vi "Format String to Numeric.vi"(0 "Expected String":string, 1 "Data Parameters.List":string[](array[string]), 2 "Ignore String":string, 5 "Format String":string, 7 "Endian":T1, 9 "Channel Type":T2, 11 "error in (no error)":errorcluster, 12 "Type":T3, 13 "Response":string) -> (4 "remaining string":string, 6 "Value":dbl, 15 "error out":errorcluster)   [LabVIEW 2020, in "Instrument Addon Engine.lvlib"]
uses:
  Instrument Addon Engine.lvlib
  Addon Shared/Types/Type Cast Type.ctl
  Addon Shared/Types/Data Channel Type.ctl
  Addon Shared/Types/Endian.ctl
  Addon Shared/Instrument Addon Shared.lvlib
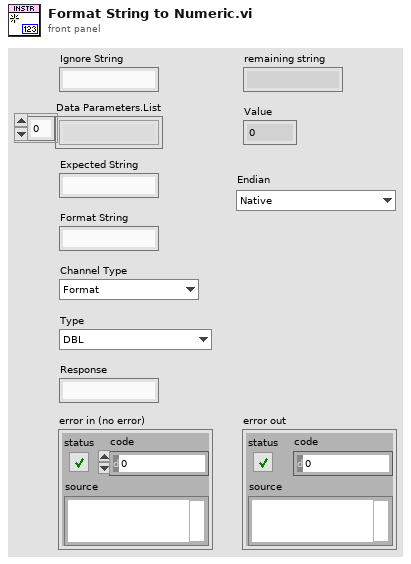
[diagram p1: front panel]
types:
  T1 = typedef "Instrument Addon Shared.lvlib/Endian.ctl" = enum16{"Native", "Little", "Big"}
  T2 = typedef "Instrument Addon Shared.lvlib/Data Channel Type.ctl" = enum16{"Format", "Comparison", "Type Cast", "Enumerated List"}
  T3 = typedef "Instrument Addon Shared.lvlib/Type Cast Type.ctl" = enum16{"DBL", "SGL", "U64", "U32", "U16", "U8", "I64", "I32", "I16", "I8"}
  T4 = enum16{"big-endian, network order", "native, host order", "little-endian"}
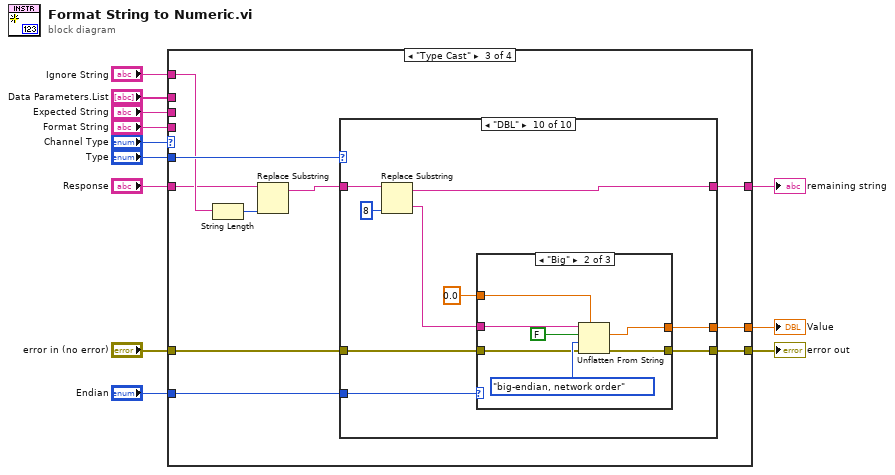
[diagram p0: block diagram]
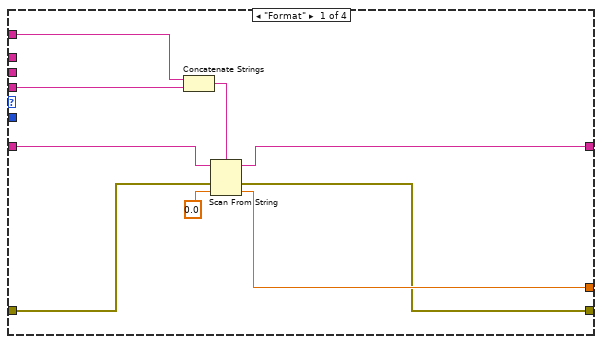
[diagram p2: hidden frame]
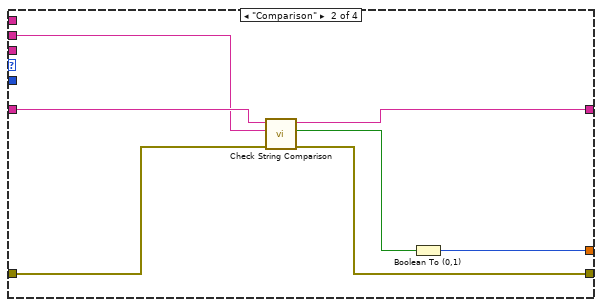
[diagram p3: hidden frame]
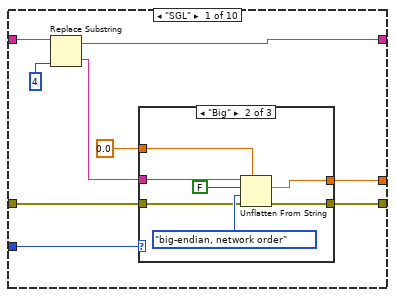
[diagram p4: hidden frame]
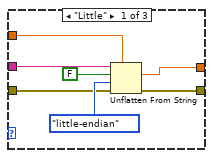
[diagram p5: hidden frame]
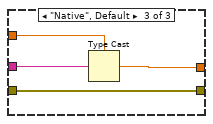
[diagram p6: hidden frame]
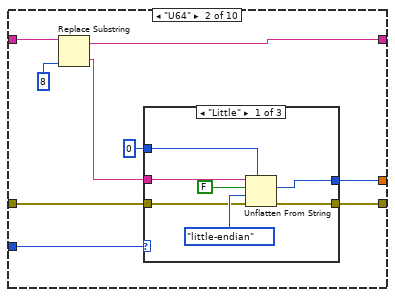
[diagram p7: hidden frame]
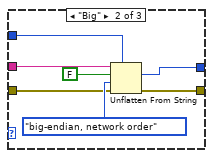
[diagram p8: hidden frame]
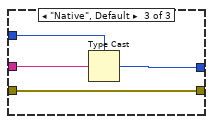
[diagram p9: hidden frame]
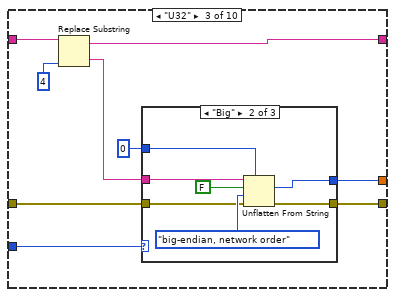
[diagram p10: hidden frame]
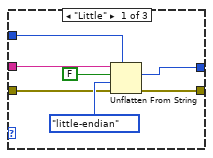
[diagram p11: hidden frame]
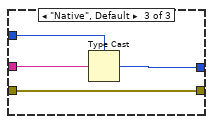
[diagram p12: hidden frame]
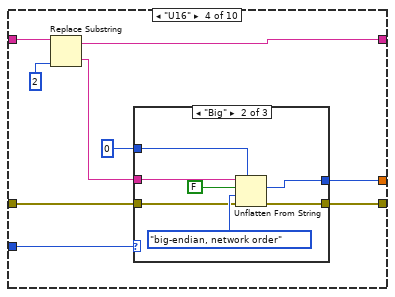
[diagram p13: hidden frame]
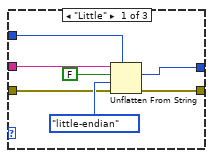
[diagram p14: hidden frame]
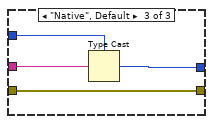
[diagram p15: hidden frame]
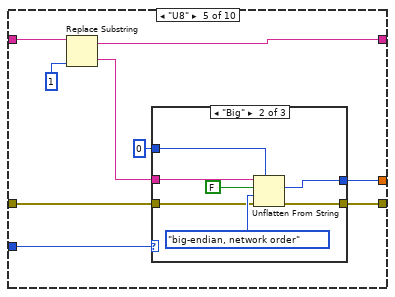
[diagram p16: hidden frame]
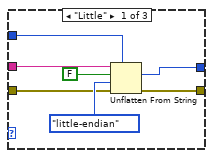
[diagram p17: hidden frame]
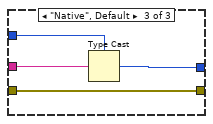
[diagram p18: hidden frame]
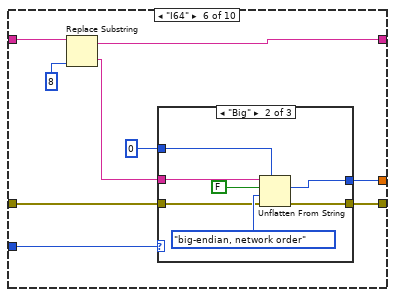
[diagram p19: hidden frame]
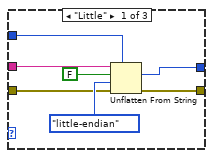
[diagram p20: hidden frame]
diagram:
  n1 = case shown="\"Type Cast\"" "Channel Type" {
    tunnel: [w20 w28 w37 w315] -> w10
    tunnel: "Response" -> [w21 w27 w34 w310]
    tunnel: [w19 w25 w38 w313] -> w4
    tunnel: "Ignore String" -> [w17 _ w35 w311]
    tunnel: "Format String" -> [w16 _ _ _]
    tunnel: "error in (no error)" -> [w15 w23 w32 w317]
    tunnel: [w14 w22 w29 w314] -> w7
    tunnel: "Expected String" -> [_ w26 _ _]
    tunnel: "Type" -> [_ _ w36 _]
    tunnel: "Data Parameters.List" -> [_ _ _ w316]
    tunnel: "Endian" -> [_ _ w30 _]
    frame "Format" {
      n2 = Concatenate Strings(w17, w16) -> (w13:string)
      n3 = Scan From String(format string=w13, input string=w21, error in=w15, default 1=0.0 ("default value 1")) -> (remaining string=w19:string, error out=w14:errorcluster, output 1=w20:dbl)  [unwired: 1 in, 1 out]
    }
    frame "Comparison" {
      n4 = call "Check String Comparison.vi"("error in (no error)"=w23, "Expected String"=w26, "String"=w27) -> ("error out"=w22:errorcluster, "Found?"=w24:bool, "string out"=w25:string)  [unwired: 6 in]
      n5 = Boolean To (0,1)(Boolean=w24) -> (0, 1=w28:i16)
    }
    frame "Type Cast" {
      n6 = String Length(string=w35) -> (length=w31:i32)
      n7 = Replace Substring(2:w31, 5:w34) -> (1:w33:string)  [unwired: 2 in, 1 out]
      n8 = case shown="\"DBL\"" w36 {
        tunnel: w33 -> [w47 w74 w101 w128 w155 w182 w209 w236 w263 w290]
        tunnel: [w46 w73 w100 w127 w154 w181 w208 w235 w262 w289] -> w38
        tunnel: [w39 w67 w93 w122 w147 w174 w202 w229 w259 w282] -> w37
        tunnel: w32 -> [w42 w70 w98 w125 w152 w179 w206 w230 w256 w287]
        tunnel: w30 -> [w41 w66 w95 w124 w151 w178 w201 w228 w258 w285]
        tunnel: [w40 w71 w94 w123 w148 w175 w203 w233 w255 w286] -> w29
        frame "SGL" {
          n9 = Replace Substring(2:4 ("length (len. of substring)"), 5:w47) -> (0:w44:string, 1:w46:string)  [unwired: 2 in]
          n10 = case shown="\"Big\"" w41 {
            tunnel: w44 -> [w54 w61 w65]
            tunnel: [w50 w57 w64] -> w39
            tunnel: sgl 0.0 -> [w51 w58 w63]
            tunnel: w42 -> [w49 w56 w62]
            tunnel: [w48 w55 w62] -> w40
            frame "Little" {
              n11 = Unflatten From String(type=w51, binary string=w54, data includes array or string size? (T)=FALSE, byte order (0:big-endian, network order)=T4."little-endian", error in (no error)=w49) -> (value=w50:sgl, error out=w48:errorcluster)  [unwired: 1 out]
            }
            frame "Big" {
              n12 = Unflatten From String(type=w58, binary string=w61, data includes array or string size? (T)=FALSE, byte order (0:big-endian, network order)=T4."big-endian, network order", error in (no error)=w56) -> (value=w57:sgl, error out=w55:errorcluster)  [unwired: 1 out]
            }
            frame "Native", Default {
              n13 = Type Cast(type=w63, x=w65) -> (*(type *) &x=w64:sgl)
            }
          }
        }
        frame "U64" {
          n14 = Replace Substring(2:8 ("length (len. of substring)"), 5:w74) -> (0:w69:string, 1:w73:string)  [unwired: 2 in]
          n15 = case shown="\"Little\"" w66 {
            tunnel: w69 -> [w81 w88 w92]
            tunnel: [w77 w84 w91] -> w67
            tunnel: u64 0 -> [w78 w85 w90]
            tunnel: w70 -> [w76 w83 w89]
            tunnel: [w75 w82 w89] -> w71
            frame "Little" {
              n16 = Unflatten From String(type=w78, binary string=w81, data includes array or string size? (T)=FALSE, byte order (0:big-endian, network order)=T4."little-endian", error in (no error)=w76) -> (value=w77:u64, error out=w75:errorcluster)  [unwired: 1 out]
            }
            frame "Big" {
              n17 = Unflatten From String(type=w85, binary string=w88, data includes array or string size? (T)=FALSE, byte order (0:big-endian, network order)=T4."big-endian, network order", error in (no error)=w83) -> (value=w84:u64, error out=w82:errorcluster)  [unwired: 1 out]
            }
            frame "Native", Default {
              n18 = Type Cast(type=w90, x=w92) -> (*(type *) &x=w91:u64)
            }
          }
        }
        frame "U32" {
          n19 = Replace Substring(2:4 ("length (len. of substring)"), 5:w101) -> (0:w97:string, 1:w100:string)  [unwired: 2 in]
          n20 = case shown="\"Big\"" w95 {
            tunnel: w97 -> [w108 w115 w119]
            tunnel: [w104 w111 w118] -> w93
            tunnel: u32 0 -> [w105 w112 w117]
            tunnel: w98 -> [w103 w110 w116]
            tunnel: [w102 w109 w116] -> w94
            frame "Little" {
              n21 = Unflatten From String(type=w105, binary string=w108, data includes array or string size? (T)=FALSE, byte order (0:big-endian, network order)=T4."little-endian", error in (no error)=w103) -> (value=w104:u32, error out=w102:errorcluster)  [unwired: 1 out]
            }
            frame "Big" {
              n22 = Unflatten From String(type=w112, binary string=w115, data includes array or string size? (T)=FALSE, byte order (0:big-endian, network order)=T4."big-endian, network order", error in (no error)=w110) -> (value=w111:u32, error out=w109:errorcluster)  [unwired: 1 out]
            }
            frame "Native", Default {
              n23 = Type Cast(type=w117, x=w119) -> (*(type *) &x=w118:u32)
            }
          }
        }
        frame "U16" {
          n24 = Replace Substring(2:2 ("length (len. of substring)"), 5:w128) -> (0:w120:string, 1:w127:string)  [unwired: 2 in]
          n25 = case shown="\"Big\"" w124 {
            tunnel: w120 -> [w135 w142 w146]
            tunnel: [w131 w138 w145] -> w122
            tunnel: u16 0 -> [w132 w139 w144]
            tunnel: w125 -> [w130 w137 w143]
            tunnel: [w129 w136 w143] -> w123
            frame "Little" {
              n26 = Unflatten From String(type=w132, binary string=w135, data includes array or string size? (T)=FALSE, byte order (0:big-endian, network order)=T4."little-endian", error in (no error)=w130) -> (value=w131:u16, error out=w129:errorcluster)  [unwired: 1 out]
            }
            frame "Big" {
              n27 = Unflatten From String(type=w139, binary string=w142, data includes array or string size? (T)=FALSE, byte order (0:big-endian, network order)=T4."big-endian, network order", error in (no error)=w137) -> (value=w138:u16, error out=w136:errorcluster)  [unwired: 1 out]
            }
            frame "Native", Default {
              n28 = Type Cast(type=w144, x=w146) -> (*(type *) &x=w145:u16)
            }
          }
        }
        frame "U8" {
          n29 = Replace Substring(2:1 ("length (len. of substring)"), 5:w155) -> (0:w150:string, 1:w154:string)  [unwired: 2 in]
          n30 = case shown="\"Big\"" w151 {
            tunnel: w150 -> [w162 w169 w173]
            tunnel: [w158 w165 w172] -> w147
            tunnel: u8 0 -> [w159 w166 w171]
            tunnel: w152 -> [w157 w164 w170]
            tunnel: [w156 w163 w170] -> w148
            frame "Little" {
              n31 = Unflatten From String(type=w159, binary string=w162, data includes array or string size? (T)=FALSE, byte order (0:big-endian, network order)=T4."little-endian", error in (no error)=w157) -> (value=w158:u8, error out=w156:errorcluster)  [unwired: 1 out]
            }
            frame "Big" {
              n32 = Unflatten From String(type=w166, binary string=w169, data includes array or string size? (T)=FALSE, byte order (0:big-endian, network order)=T4."big-endian, network order", error in (no error)=w164) -> (value=w165:u8, error out=w163:errorcluster)  [unwired: 1 out]
            }
            frame "Native", Default {
              n33 = Type Cast(type=w171, x=w173) -> (*(type *) &x=w172:u8)
            }
          }
        }
        frame "I64" {
          n34 = Replace Substring(2:8 ("length (len. of substring)"), 5:w182) -> (0:w177:string, 1:w181:string)  [unwired: 2 in]
          n35 = case shown="\"Big\"" w178 {
            tunnel: w177 -> [w189 w196 w200]
            tunnel: [w185 w192 w199] -> w174
            tunnel: i64 0 -> [w186 w193 w198]
            tunnel: w179 -> [w184 w191 w197]
            tunnel: [w183 w190 w197] -> w175
            frame "Little" {
              n36 = Unflatten From String(type=w186, binary string=w189, data includes array or string size? (T)=FALSE, byte order (0:big-endian, network order)=T4."little-endian", error in (no error)=w184) -> (value=w185:i64, error out=w183:errorcluster)  [unwired: 1 out]
            }
            frame "Big" {
              n37 = Unflatten From String(type=w193, binary string=w196, data includes array or string size? (T)=FALSE, byte order (0:big-endian, network order)=T4."big-endian, network order", error in (no error)=w191) -> (value=w192:i64, error out=w190:errorcluster)  [unwired: 1 out]
            }
            frame "Native", Default {
              n38 = Type Cast(type=w198, x=w200) -> (*(type *) &x=w199:i64)
            }
          }
        }
        frame "I32" {
          n39 = Replace Substring(2:4 ("length (len. of substring)"), 5:w209) -> (0:w205:string, 1:w208:string)  [unwired: 2 in]
          n40 = case shown="\"Native\", Default" w201 {
            tunnel: w205 -> [w216 w223 w227]
            tunnel: [w212 w219 w226] -> w202
            tunnel: 0 -> [w213 w220 w225]
            tunnel: w206 -> [w211 w218 w224]
            tunnel: [w210 w217 w224] -> w203
            frame "Little" {
              n41 = Unflatten From String(type=w213, binary string=w216, data includes array or string size? (T)=FALSE, byte order (0:big-endian, network order)=T4."little-endian", error in (no error)=w211) -> (value=w212:i32, error out=w210:errorcluster)  [unwired: 1 out]
            }
            frame "Big" {
              n42 = Unflatten From String(type=w220, binary string=w223, data includes array or string size? (T)=FALSE, byte order (0:big-endian, network order)=T4."big-endian, network order", error in (no error)=w218) -> (value=w219:i32, error out=w217:errorcluster)  [unwired: 1 out]
            }
            frame "Native", Default {
              n43 = Type Cast(type=w225, x=w227) -> (*(type *) &x=w226:i32)
            }
          }
        }
        frame "I16" {
          n44 = Replace Substring(2:2 ("length (len. of substring)"), 5:w236) -> (0:w231:string, 1:w235:string)  [unwired: 2 in]
          n45 = case shown="\"Big\"" w228 {
            tunnel: w231 -> [w243 w250 w254]
            tunnel: [w239 w246 w253] -> w229
            tunnel: i16 0 -> [w240 w247 w252]
            tunnel: w230 -> [w238 w245 w251]
            tunnel: [w237 w244 w251] -> w233
            frame "Little" {
              n46 = Unflatten From String(type=w240, binary string=w243, data includes array or string size? (T)=FALSE, byte order (0:big-endian, network order)=T4."little-endian", error in (no error)=w238) -> (value=w239:i16, error out=w237:errorcluster)  [unwired: 1 out]
            }
            frame "Big" {
              n47 = Unflatten From String(type=w247, binary string=w250, data includes array or string size? (T)=FALSE, byte order (0:big-endian, network order)=T4."big-endian, network order", error in (no error)=w245) -> (value=w246:i16, error out=w244:errorcluster)  [unwired: 1 out]
            }
            frame "Native", Default {
              n48 = Type Cast(type=w252, x=w254) -> (*(type *) &x=w253:i16)
            }
          }
        }
        frame "I8" {
          n49 = Replace Substring(2:1 ("length (len. of substring)"), 5:w263) -> (0:w260:string, 1:w262:string)  [unwired: 2 in]
          n50 = case shown="\"Big\"" w258 {
            tunnel: w260 -> [w270 w277 w281]
            tunnel: [w266 w273 w280] -> w259
            tunnel: i8 0 -> [w267 w274 w279]
            tunnel: w256 -> [w265 w272 w278]
            tunnel: [w264 w271 w278] -> w255
            frame "Little" {
              n51 = Unflatten From String(type=w267, binary string=w270, data includes array or string size? (T)=FALSE, byte order (0:big-endian, network order)=T4."little-endian", error in (no error)=w265) -> (value=w266:i8, error out=w264:errorcluster)  [unwired: 1 out]
            }
            frame "Big" {
              n52 = Unflatten From String(type=w274, binary string=w277, data includes array or string size? (T)=FALSE, byte order (0:big-endian, network order)=T4."big-endian, network order", error in (no error)=w272) -> (value=w273:i8, error out=w271:errorcluster)  [unwired: 1 out]
            }
            frame "Native", Default {
              n53 = Type Cast(type=w279, x=w281) -> (*(type *) &x=w280:i8)
            }
          }
        }
        frame "DBL" {
          n54 = Replace Substring(2:8 ("length (len. of substring)"), 5:w290) -> (0:w284:string, 1:w289:string)  [unwired: 2 in]
          n55 = case shown="\"Big\"" w285 {
            tunnel: w284 -> [w297 w304 w308]
            tunnel: [w293 w300 w307] -> w282
            tunnel: 0.0 -> [w294 w301 w306]
            tunnel: w287 -> [w292 w299 w305]
            tunnel: [w291 w298 w305] -> w286
            frame "Little" {
              n56 = Unflatten From String(type=w294, binary string=w297, data includes array or string size? (T)=FALSE, byte order (0:big-endian, network order)=T4."little-endian", error in (no error)=w292) -> (value=w293:dbl, error out=w291:errorcluster)  [unwired: 1 out]
            }
            frame "Big" {
              n57 = Unflatten From String(type=w301, binary string=w304, data includes array or string size? (T)=FALSE, byte order (0:big-endian, network order)=T4."big-endian, network order", error in (no error)=w299) -> (value=w300:dbl, error out=w298:errorcluster)  [unwired: 1 out]
            }
            frame "Native", Default {
              n58 = Type Cast(type=w306, x=w308) -> (*(type *) &x=w307:dbl)
            }
          }
        }
      }
    }
    frame "Enumerated List" {
      n59 = String Length(string=w311) -> (length=w312:i32)
      n60 = Replace Substring(2:w312, 5:w310) -> (1:w309:string)  [unwired: 2 in, 1 out]
      n61 = for {
        shift-right: [w325] -> w314
        shift-left: w317 -> [w325]
        tunnel: w316 -> [w329] mode=indexing
        tunnel: w309 -> [w320]
        tunnel: [w326] -> w315
        tunnel: [w318] -> w313
        i -> [w328]
        stop <- w321 stop-if-true
        n62 = String Length(string=w329) -> (length=w324:i32)
        n63 = Replace Substring(2:w324, 3:0 ("offset (0)"), 5:w320) -> (0:w322:string, 1:w319:string)  [unwired: 1 in]
        n64 = Equal?(x=w322, y=w329) -> (x = y?=w321:bool)
        n65 = Select(t=w319, s=w321, f=w320) -> (s? t:f=w318:string)
        n66 = Select(t=w328, s=w321, f=-1) -> (s? t:f=w326:i32)
      }
    }
  }
  "Value" <- w10
  "error out" <- w7
  "remaining string" <- w4
